vi "Validate_Do.vi"(8 "error in (no error)":errorcluster, 11 "Project Action Interface in":refnum<class "Project Action Interface.lvclass">) -> (0 "error out":errorcluster, 1 "Valid?":bool, 3 "Project Action Interface out":refnum<class "Project Action Interface.lvclass">)   [LabVIEW 2020, in "ProjectBuilder.lvlib" / "Project Action Interface.lvclass"]
uses:
  Project Action Interface.lvclass
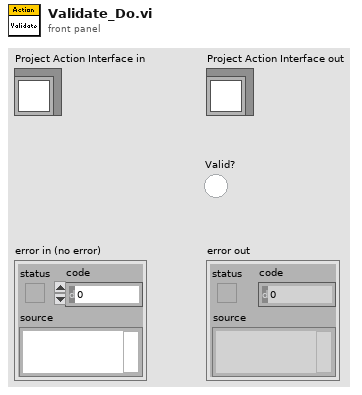
[diagram p1: front panel]
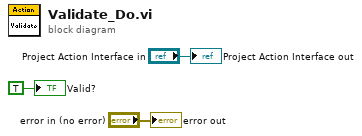
[diagram p0: block diagram]
diagram:
  "error out" <- "error in (no error)"
  "Project Action Interface out" <- "Project Action Interface in"
  "Valid?" <- TRUE
